vi "Add Rx Monitor Status Section.vi"(8 "error in":errorcluster, 11 "Section ref in":T1 format="%.0x") -> (0 "error out":errorcluster, 1 "Monitor Queue Status channel Refs":T1[](array[typedef]) format="%.0x", 2 "Monitor Queue Status Section Ref out":T1 format="%.0x", 3 "Section Ref out":T1 format="%.0x")   [LabVIEW 2020, in "AIM ARINC 664 Scripting.lvlib"]
uses:
  AIM ARINC 664 Scripting.lvlib
  <vilib>/NI VeriStand/Custom Device API/Custom Device Item Ref.ctl
  Controls/RxStatus Enum.ctl
  Constants.vi
  <vilib>/NI VeriStand/Custom Device API/Custom Device API.lvlib
  <vilib>/NI VeriStand/Custom Device API/Custom Device Channel Type.ctl
  <vilib>/NI VeriStand/Custom Device API/Custom Device Channel.ctl
  <vilib>/Utility/Data Type/NI_Data Type.lvlib
  <vilib>/NI/NI VeriStand Advanced SysDef API/SysDef API/Advanced System Definition.lvlib
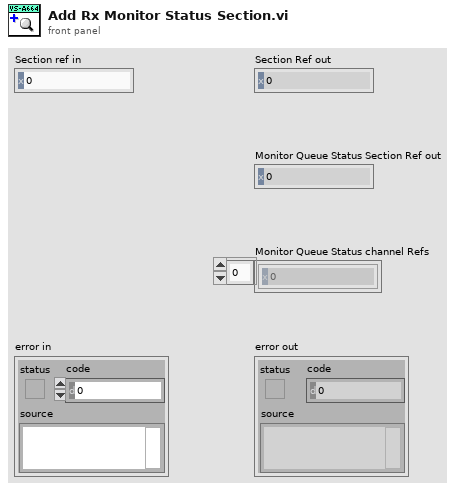
[diagram p1: front panel]
types:
  T1 = typedef "Custom Device API.lvlib/Custom Device Item Ref.ctl" = u64
  T2 = enum16{"FDX_MON_STAT_EMPTY", "FDX_MON_STAT_FILLED", "FDX_MON_STAT_FULL", "FDX_MON_STAT_OVERFLOW", "FDX_MON_STAT_ERROR"}
  T3 = typedef "RxStatus Enum.ctl" = enum16{"FDX_STAT_STOP", "FDX_STAT_RUN", "FDX_STAT_ERROR"}
  T4 = typedef "Custom Device API.lvlib/Custom Device Channel.ctl" = cluster{"Type":T5, "Units":string, "Default Value":dbl, "Faultable":bool, "Scalable":bool}
  T5 = typedef "Custom Device API.lvlib/Custom Device Channel Type.ctl" = enum16{"Input", "Output"}
  T6 = cluster{"Monitor QueueStatus Channel":string, "enum names":string[], "Values":dbl[]}
  T7 = cluster{"Monitor RxStatus Channel":string, "enum names":string[], "Values":dbl[]}
  T8 = cluster{"Monitor RxStatus Channel":string, "enum names":string[], "Values":dbl[]}[]
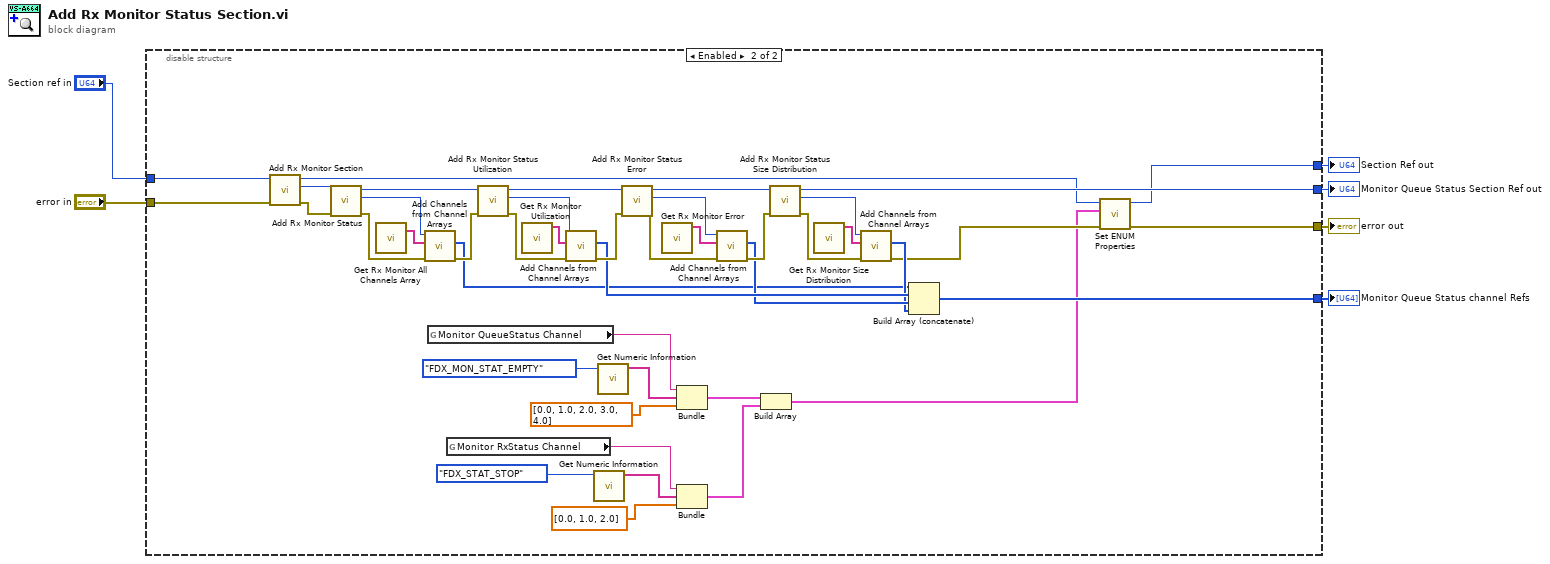
[diagram p0: block diagram]
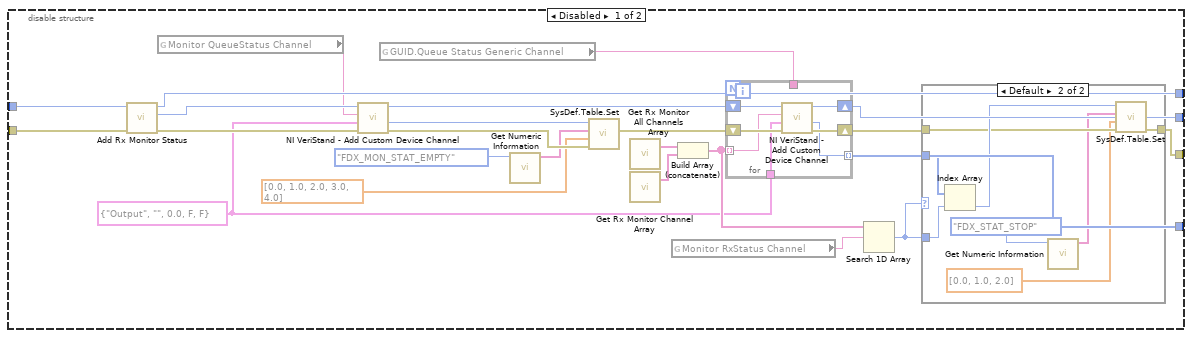
[diagram p2: hidden frame]
diagram:
  n1 = disable-structure shown="Enabled" {
    disable-tunnel: "Section ref in" -> [w30 w89]
    disable-tunnel: "error in" -> [w29 w88]
    disable-tunnel: [w27 w66] -> w4
    disable-tunnel: [w26 w55] -> w3
    disable-tunnel: [w11 w71] -> w2
    disable-tunnel: [w8 w64] -> w1
    frame Disabled {
      w7 = T4 {"Type"=enum."Output", "Units"="", "Default Value"=0.0, "Faultable"=FALSE, "Scalable"=FALSE} ("Channel")
      n2 = call "Add Rx Monitor Status.vi"("error in (no error)"=w29, "Section ref in"=w30) -> ("error out"=w28:errorcluster, "Section Ptr"=w25:T1, "Parent Ref out"=w26:T1)  [unwired: 7 in]
      n3 = global read "Constants.vi" "Monitor QueueStatus Channel"() -> (w24:string)
      n4 = call <vilib>:"NI VeriStand - Add Custom Device Channel.vi"("error in (no error)"=w28, "Channel"=w7, "Channel Name"=w24, "Parent Ref in"=w25) -> ("error out"=w21:errorcluster, "Channel Ref"=w19:T1, "Parent Ref out"=w22:T1)  [unwired: 4 in, 1 out]
      n5 = global read "Constants.vi" "GUID.Queue Status Generic Channel"() -> (w23:string)
      n6 = call <vilib>:"Get Numeric Information.vi"("variant"=T2."FDX_MON_STAT_EMPTY" ("Enum")) -> ("enum names"=w18:string[])  [unwired: 7 in, 3 out]
      n7 = call <vilib>:"SysDef.Table.Set.vi"("error in (no error)"=w21, "Values"=dbl[] [0.0, 1.0, 2.0, 3.0, 4.0], "Names"=w18, "nodeID"=w19) -> ("error out"=w20:errorcluster)  [unwired: 6 in, 1 out]
      n8 = call "Get Rx Monitor All Channels Array.vi"() -> ("Channel Array"=w15:string[])  [unwired: 3 in]
      n9 = call "Get Rx Monitor Channel Array.vi"() -> ("Channel Array"=w14:string[])  [unwired: 3 in]
      n10 = global read "Constants.vi" "Monitor RxStatus Channel"() -> (w13:string)
      n11 = Build Array (concatenate)(w15, w14) -> (w12:string[])
      n12 = for {
        tunnel: [w42] -> w11 mode=indexing
        shift-right: [w43] -> w9
        shift-left: w20 -> [w46]
        tunnel: w12 -> [w40] mode=indexing
        tunnel: w7 -> [w41]
        tunnel: w23 -> [_]
        shift-right: [w45] -> w27
        shift-left: w22 -> [w44]
        n13 = call <vilib>:"NI VeriStand - Add Custom Device Channel.vi"("error in (no error)"=w46, "Channel"=w41, "Channel Name"=w40, "Parent Ref in"=w44) -> ("error out"=w43:errorcluster, "Channel Ref"=w42:T1, "Parent Ref out"=w45:T1)  [unwired: 4 in, 1 out]
      }
      n14 = Search 1D Array(1D array=w12, element=w13) -> (index of element=w10:i32)  [unwired: 1 in]
      n15 = case shown="Default" w10 {
        tunnel: w11 -> [_ w39]
        tunnel: w10 -> [_ w38]
        tunnel: w9 -> [w31 w36]
        tunnel: [w31 w35] -> w8
        frame -1 {
        }
        frame Default {
          n16 = Index Array(array=w39, index=w38) -> (element=w37:T1)
          n17 = call <vilib>:"Get Numeric Information.vi"("variant"=RxStatus_Enum."FDX_STAT_STOP" ("Enum")) -> ("enum names"=w33:string[])  [unwired: 7 in, 3 out]
          n18 = call <vilib>:"SysDef.Table.Set.vi"("error in (no error)"=w36, "Values"=dbl[] [0.0, 1.0, 2.0], "Names"=w33, "nodeID"=w37) -> ("error out"=w35:errorcluster)  [unwired: 6 in, 1 out]
        }
      }
    }
    frame Enabled {
      n19 = call "Add Rx Monitor Section.vi"("error in (no error)"=w88, "Section ref in"=w89) -> ("error out"=w51:errorcluster, "Section Ptr"=w54:T1, "Parent Ref out"=w56:T1)  [unwired: 7 in]
      n20 = call "Add Rx Monitor Status.vi"("error in (no error)"=w51, "Section ref in"=w54) -> ("error out"=w50:errorcluster, "Section Ptr"=w53:T1, "Parent Ref out"=w52:T1)  [unwired: 7 in]
      n21 = call "Get Rx Monitor All Channels Array.vi"() -> ("Channel Array"=w69:string[])  [unwired: 3 in]
      n22 = call "Add Channels from Channel Arrays.vi"("error in"=w50, "Channel Array"=w69, "Section Ptr in"=w53) -> ("error out"=w70:errorcluster, "Channel Refs"=w49:T1[])  [unwired: 6 in, 1 out]
      n23 = global read "Constants.vi" "Monitor QueueStatus Channel"() -> (w47:string)
      n24 = global read "Constants.vi" "Monitor RxStatus Channel"() -> (w48:string)
      n25 = call "Add Rx Monitor Status Utilization.vi"("error in (no error)"=w70, "Section ref in"=w52) -> ("error out"=w76:errorcluster, "Section Ptr"=w75:T1, "Parent Ref out"=w78:T1)  [unwired: 7 in]
      n26 = call "Get Rx Monitor Utilization.vi"() -> ("Channel Array"=w77:string[])  [unwired: 11 in]
      n27 = call "Add Channels from Channel Arrays.vi"("error in"=w76, "Channel Array"=w77, "Section Ptr in"=w75) -> ("error out"=w79:errorcluster, "Channel Refs"=w74:T1[])  [unwired: 6 in, 1 out]
      n28 = call <vilib>:"Get Numeric Information.vi"("variant"=RxStatus_Enum."FDX_STAT_STOP" ("Enum")) -> ("enum names"=w60:string[])  [unwired: 7 in, 3 out]
      n29 = call <vilib>:"Get Numeric Information.vi"("variant"=T2."FDX_MON_STAT_EMPTY" ("Enum")) -> ("enum names"=w63:string[])  [unwired: 7 in, 3 out]
      n30 = call "Add Rx Monitor Status Error.vi"("error in (no error)"=w79, "Section ref in"=w78) -> ("error out"=w83:errorcluster, "Section Ptr"=w80:T1, "Parent Ref out"=w85:T1)  [unwired: 7 in]
      n31 = call "Get Rx Monitor Error.vi"() -> ("Channel Array"=w87:string[])  [unwired: 11 in]
      n32 = Bundle("Monitor QueueStatus Channel"=w47, "enum names"=w63, "Values"=dbl[] [0.0, 1.0, 2.0, 3.0, 4.0]) -> (w58:T6)  [unwired: 1 in]
      n33 = Bundle("Monitor RxStatus Channel"=w48, "enum names"=w60, "Values"=dbl[] [0.0, 1.0, 2.0]) -> (w59:T7)  [unwired: 1 in]
      n34 = call "Add Channels from Channel Arrays.vi"("error in"=w83, "Channel Array"=w87, "Section Ptr in"=w80) -> ("error out"=w84:errorcluster, "Channel Refs"=w73:T1[])  [unwired: 6 in, 1 out]
      n35 = Build Array(w58, w59) -> (w57:T8)
      n36 = call "Add Rx Monitor Status Size Distribution.vi"("error in (no error)"=w84, "Section ref in"=w85) -> ("error out"=w81:errorcluster, "Section Ptr"=w82:T1, "Parent Ref out"=w66:T1)  [unwired: 7 in]
      n37 = call "Get Rx Monitor Size Distribution.vi"() -> ("Channel Array"=w86:string[])  [unwired: 11 in]
      n38 = call "Add Channels from Channel Arrays.vi"("error in"=w81, "Channel Array"=w86, "Section Ptr in"=w82) -> ("error out"=w65:errorcluster, "Channel Refs"=w72:T1[])  [unwired: 6 in, 1 out]
      n39 = Build Array (concatenate)(w49, w74, w73, w72) -> (w71:T1[])
      n40 = call "Set ENUM Properties.vi"("error in"=w65, "enum to be changes"=w57, "parent ref in"=w56) -> ("error out"=w64:errorcluster, "parent ref out"=w55:T1)  [unwired: 7 in]
    }
  }
  "Monitor Queue Status Section Ref out" <- w4
  "Section Ref out" <- w3
  "error out" <- w1
  "Monitor Queue Status channel Refs" <- w2
